vi "rad_Find App Img File.vi"(8 "Error In":errorcluster, 11 "Temp Image Path":path) -> (0 "Error Out":errorcluster, 3 "LVAppImg Path":path)   [LabVIEW 2023]
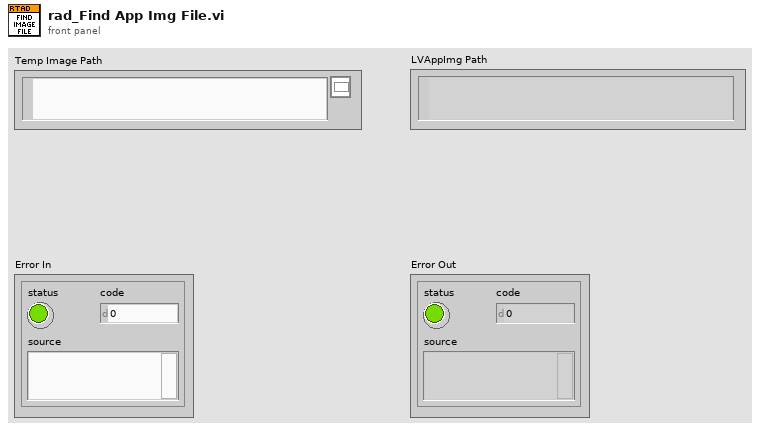
[diagram p1: front panel]
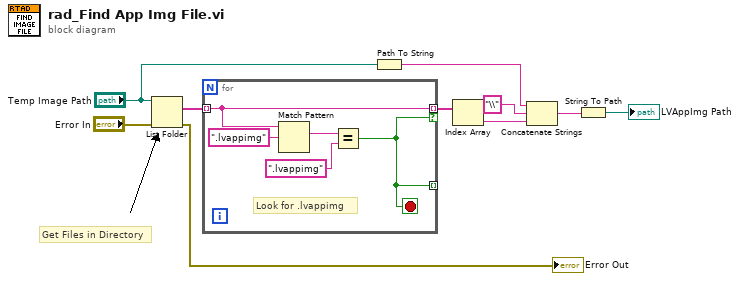
[diagram p0: block diagram]
diagram:
  # "Get Files in Directory"
  n1 = List Folder(path="Temp Image Path", error in="Error In") -> (filenames=w9:string[], error out=→"Error Out":errorcluster)  [unwired: 2 in, 2 out]
  n2 = for {
    tunnel: w9 -> [w12] mode=indexing
    tunnel: [w12] -> w8 mode=indexing if=w11
    tunnel: [w11] -> _ mode=indexing
    stop <- w11 stop-if-true
    # "Look for .lvappimg"
    n3 = Match Pattern(string=w12, regular expression=".lvappimg") -> (match substring=w14:string)  [unwired: 1 in, 3 out]
    n4 = Equal?(x=w14, y=".lvappimg") -> (x = y?=w11:bool)
  }
  n5 = Path To String(path="Temp Image Path") -> (string=w3:string)
  n6 = Index Array(array=w8) -> (element=w7:string)  [unwired: 1 in]
  n7 = Concatenate Strings(w3, "\\" ("string"), w7) -> (w2:string)
  n8 = String To Path(string=w2) -> (path=→"LVAppImg Path":path)
